vi "getOperationMode.vi"(8 "error in (no error)":errorcluster, 11 "IComponent in":refnum<class "IComponent.lvclass">) -> (0 "error out":errorcluster, 2 "OperationMode out":T1 items=["daqOperationModeTypeUnknown", "daqOperationModeTypeIdle", "daqOperationModeTypeOperation", "daqOperationModeTypeSafeOperation"], 3 "IComponent out":refnum<class "IComponent.lvclass">)   [LabVIEW 2022 SP3, in "openDAQ.lvlib" / "IBaseObject.lvlib" / "IPropertyObject.lvlib" / "IComponent.lvlib" / "IComponent.lvclass"]
uses:
  <instrlib>/openDAQ/Public/Classes/IComponent/IComponent.lvclass
  <instrlib>/openDAQ/Public/Classes/IComponent/IComponent.lvclass/IComponent.ctl
  <instrlib>/openDAQ/Binaries/Windows/x86/copendaq32.dll
  <instrlib>/openDAQ/Public/TypeDef/daqOperationModeType.ctl
  <instrlib>/openDAQ/openDAQ.lvlib
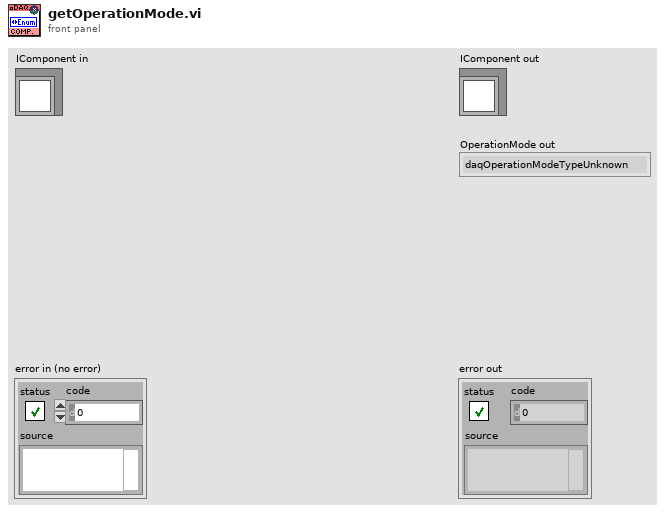
[diagram p1: front panel]
types:
  T1 = typedef "openDAQ.lvlib/daqOperationModeType.ctl" = u16
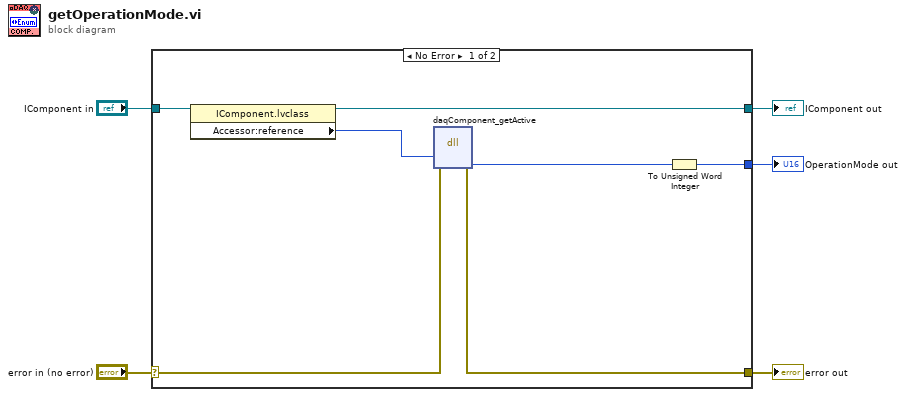
[diagram p0: block diagram]
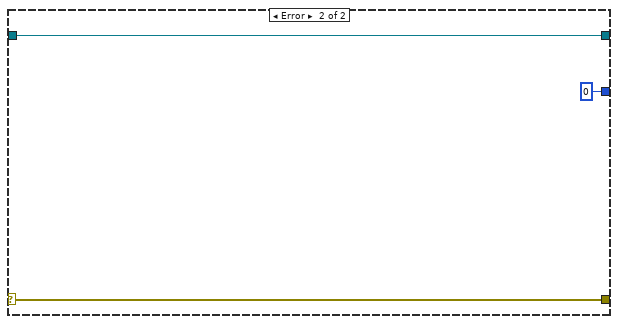
[diagram p2: hidden frame]
diagram:
  n1 = case shown="No Error" "error in (no error)" {
    selector: "error in (no error)" -> [w8 w15]
    tunnel: [w9 w15] -> w4
    tunnel: [w11 w14] -> w2
    tunnel: "IComponent in" -> [w12 w14]
    tunnel: [w6 u16 0] -> w1
    frame No Error {
      n2 = property class="IComponent.lvclass"(reference=w12) -> (reference out=w11:refnum<class "IComponent.lvclass">, "Accessor:reference"=w10:i64)  [unwired: 1 in, 1 out]
      n3 = dll-call lib="C:/Program Files (x86)/National Instruments/LabVIEW 2022/instr.lib/openDAQ/Binaries/Windows/x86/copendaq*.*" fn="daqComponent_getActive"(error in=w8, "component"=w10) -> (error out=w9:errorcluster, "active"=w7:i64)  [unwired: 5 in, 1 out]
      n4 = To Unsigned Word Integer(number=w7) -> (unsigned 16bit integer=w6:u16)
    }
    frame Error {
    }
  }
  "error out" <- w4
  "IComponent out" <- w2
  "OperationMode out" <- w1
